vi "P-541 Get Value.vi"(0 "VISA Pass Thru":refnum<visa-resource-name>, 7 "Cmd Reply":string, 11 "Error In":errorcluster) -> (4 "VISA Ref Dup":refnum<visa-resource-name>, 8 "Bool":bool, 10 "Value":dbl, 15 "Error Out":errorcluster)   [LabVIEW 2020]
uses:
  <vilib>/Utility/error.llb/whitespace.ctl
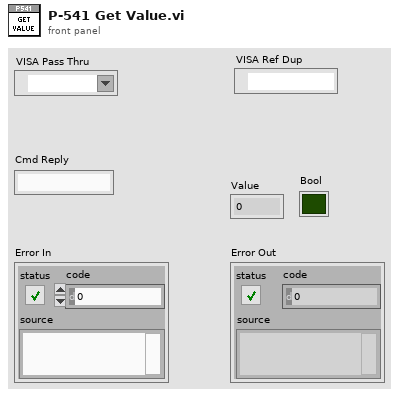
[diagram p1: front panel]
types:
  T1 = typedef "whitespace.ctl" = u16
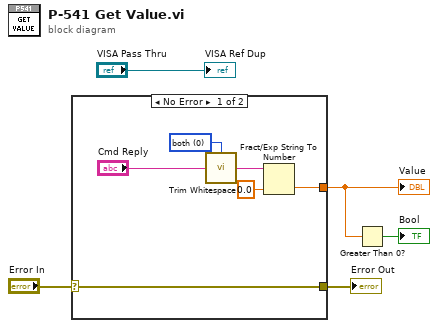
[diagram p0: block diagram]
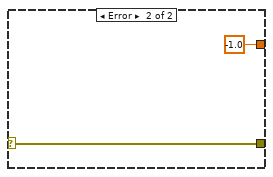
[diagram p2: hidden frame]
diagram:
  n1 = case shown="No Error" "Error In" {
    selector: "Error In" -> [w8 w13]
    tunnel: [w8 w13] -> w5
    tunnel: [w7 -1.0] -> w4
    frame No Error {
      w11 = T1 0 items=["both", "start of string", "end of string"] ("location (both)")
      n2 = call <vilib>:"Trim Whitespace.vi"("string"="Cmd Reply", "location (both)"=w11) -> ("trimmed string"=w10:string)
      n3 = Fract/Exp String To Number(string=w10, default (0 dbl)=0.0 ("default (0 DBL)")) -> (number=w7:dbl)  [unwired: 2 in, 1 out]
    }
    frame Error {
    }
  }
  "Value" <- w4
  "Error Out" <- w5
  n4 = Greater Than 0?(x=w4) -> (x > 0?=→"Bool":bool)
  "VISA Ref Dup" <- "VISA Pass Thru"
